vi "gmmregRegistrationLowLevel.vi"(0 "nctrlpts":i32, 1 "coordCtrlPts":dbl[](array[numeric]), 2 "npts":i32, 3 "coord":dbl[](array[numeric]), 4 "nptsScene":i32, 5 "coordScene":dbl[](array[numeric]), 6 "nOut":i32, 7 "out":dbl[](array[numeric]), 8 "param0":dbl[](array[numeric]), 9 "dim (3)":i32=3, 10 "normParams":dbl[](array[numeric]), 11 "lambda":dbl[](array[numeric]), 12 "denormParams":dbl[](array[numeric]), 13 "scale":dbl[](array[numeric])) -> (14 "normParams out":dbl[](array[numeric]), 15 "scale out":dbl[](array[numeric]), 16 "denormParams out":dbl[](array[numeric]), 17 "nscale out":i32, 18 "param0 out":dbl[](array[numeric]), 19 "lambda out":dbl[](array[numeric]), 20 "nctrlpts out":i32, 21 "coordCtrlPts out":dbl[](array[numeric]), 22 "npts out":i32, 23 "coord out":dbl[](array[numeric]), 24 "nptsScene out":i32, 25 "coordScene out":dbl[](array[numeric]), 26 "nOut out":i32, 27 "out out":dbl[](array[numeric]))   [LabVIEW 2017]
uses:
  dll/wormUtilities/x64/Release/wormUtilities.dll
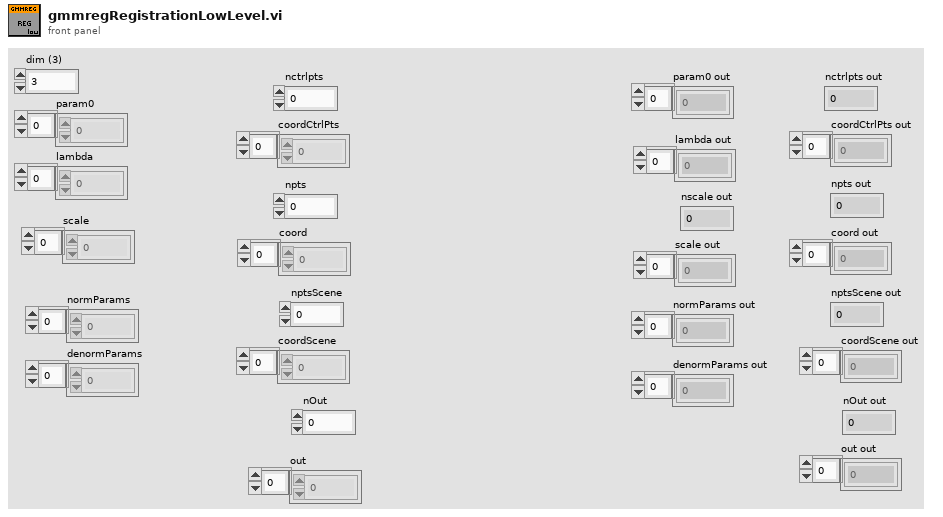
[diagram p1: front panel]
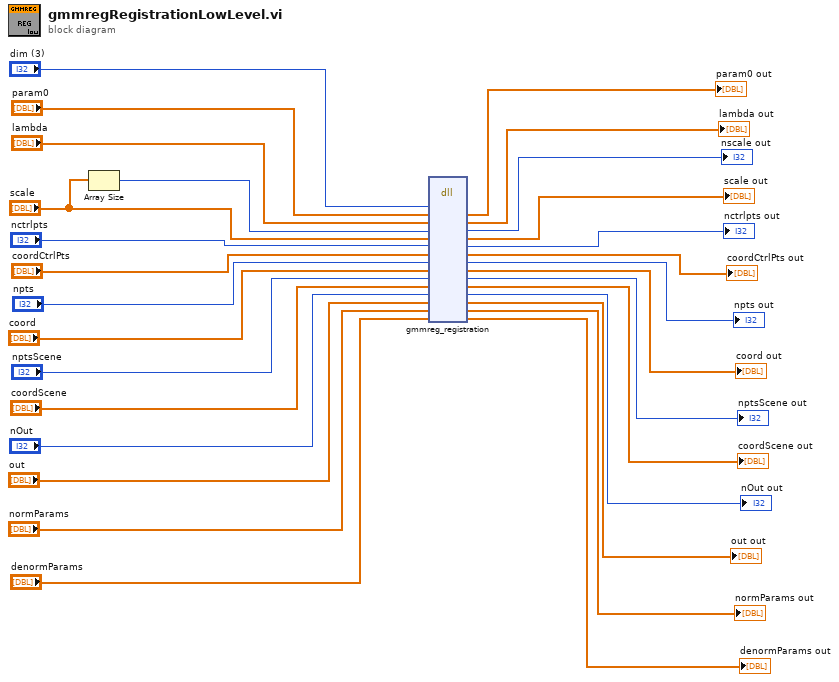
[diagram p0: block diagram]
diagram:
  n1 = Array Size(array="scale") -> (size(s)=w1:i32)
  n2 = dll-call lib="C:/Users/francesco/dev/pump-probe/dll/wormUtilities/x64/Release/wormUtilities.dll" fn="gmmreg_registration"("dim"="dim (3)", "param0"="param0", "lambda"="lambda", "nscale"=w1, "scale"="scale", "nctrlpts"="nctrlpts", "coordCtrlPts"="coordCtrlPts", "npts"="npts", "coord"="coord", "nptsScene"="nptsScene", "coordScene"="coordScene", "nOut"="nOut", "out"="out", "normParams"="normParams", "denormParams"="denormParams") -> ("param0"=→"param0 out":dbl[], "lambda"=→"lambda out":dbl[], "nscale"=→"nscale out":i32, "scale"=→"scale out":dbl[], "nctrlpts"=→"nctrlpts out":i32, "coordCtrlPts"=→"coordCtrlPts out":dbl[], "npts"=→"npts out":i32, "coord"=→"coord out":dbl[], "nptsScene"=→"nptsScene out":i32, "coordScene"=→"coordScene out":dbl[], "nOut"=→"nOut out":i32, "out"=→"out out":dbl[], "normParams"=→"normParams out":dbl[], "denormParams"=→"denormParams out":dbl[])  [unwired: 5 in, 2 out]
